vi "Sweep Control.vi"(0 "Scan control":T6=[{"Priority"=enum."Priority 1", "Scan name"=enum."OFF"}, {"Priority"=enum."Priority 0", "Scan name"=enum."Field"}, {"Priority"=enum."Priority 3", "Scan name"=enum."OFF"}, {"Priority"=enum."Priority 2", "Scan name"=enum."OFF"}], 1 "Scan parameters":T4=[{"DAQ Channel"=0, "Label"="\nappliedDC=", "Start"=-0.00372, "End"=0.00428, "Step"=5e-05, "B sweep rate"=0.0}, {"DAQ Channel"=3, "Label"="\nappliedField=", "Start"=0.3, "End"=0.0, "Step"=0.02, "B sweep rate"=0.05}, {"DAQ Channel"=3, "Label"="\nappliedVbg=", "Start"=-1.55, "End"=3.0, "Step"=0.015, "B sweep rate"=2.0}, {"DAQ Channel"=3, "Label"="\nappliedField=", "Start"=0.0, "End"=10000.0, "Step"=5000.0, "B sweep rate"=0.0}] {"B sweep rate" format="%.2f"; "Step" format="%#_6p"; "End" format="%#_6p"; "Start" format="%#_6p"}, 3 "Comments":string="B sweep from 0.3T to 0T, 0.02T step\nDC sweep from -4mV to 4mV, 5uV step\nVbg = -5V\nVsg=40mV\nT<60mK\n\nI+/-: rightwire 1/2 200uV + DC sweep, f=9\nI2-: grounded on 4\nBase f=3\nV+/-: 5/7\nV2+/-: 4/28\nVsg: 6", 4 "Experiment folder name":string="21-SmallBsweep-DCsweep-rightdrive12-leftgrounded") -> ()   [LabVIEW 2016]
uses:
  Typedefs/ScanControl.ctl
  Typedefs/Cluster - ScanControl.ctl
  Typedefs/Enum - Priority.ctl
  Typedefs/Enum - Action.ctl
  Typedefs/ScanParamters.ctl
  Typedefs/Cluster - ScanParamters.ctl
  Typedefs/PostAction.ctl
  Typedefs/Enum - PostAction.ctl
  <userlib>/_OpenG.lib/array/array.llb/Empty 1D Array (Variant)__ogtk.vi
panel:
  in  "Channels: AO":T1={"AO amp (V)"=[0.0002, 0.0, 0.0, 0.0, 0.0, 0.0, 0.0, 0.0], "AO DC (V)"=[-0.004, 0.0, 0.04, 0.0, 0.0, 0.0, 0.0, 0.0], "AO f (Hz)"=[9.0, 3.0, 3.0, 3.0, 3.0, 3.0, 3.0, 3.0], "AO phi (deg)"=[0.0, 0.0, 0.0, 0.0, 0.0, 0.0, 0.0, 0.0], "function"=[enum."Sine Wave", enum."Sine Wave", enum."Sine Wave", enum."Sine Wave", enum."Sine Wave", enum."Sine Wave", enum."Sine Wave", enum."Sine Wave"]} {"AO DC (V)" format="%#_6p"; "AO amp (V)" format="%#_6p"}
  in  "Experiment":enum16{"IV", "lockin_time", "Lockin_Vsg"}(ring)=enum."Lockin_Vsg"
  in  "Post action (indexing priority)":T2=[enum."Do Nothing", enum."Wait", enum."Do Nothing", enum."Do Nothing"]
  in  "Number of IV curves":i32=1
  # "Instructions: \n1, you can put multiple scan names in one priority.\n2 OFF has to put in last priority"
  # "if you use the lockin\nprogram remember to\nset BG/SG parameters in\n'lockin_Vsg_multichannel.vi'"
  # "0"
  # "1"
  # "2"
  # "3"
  # "4"
  # "5"
  # "6"
  # "7"
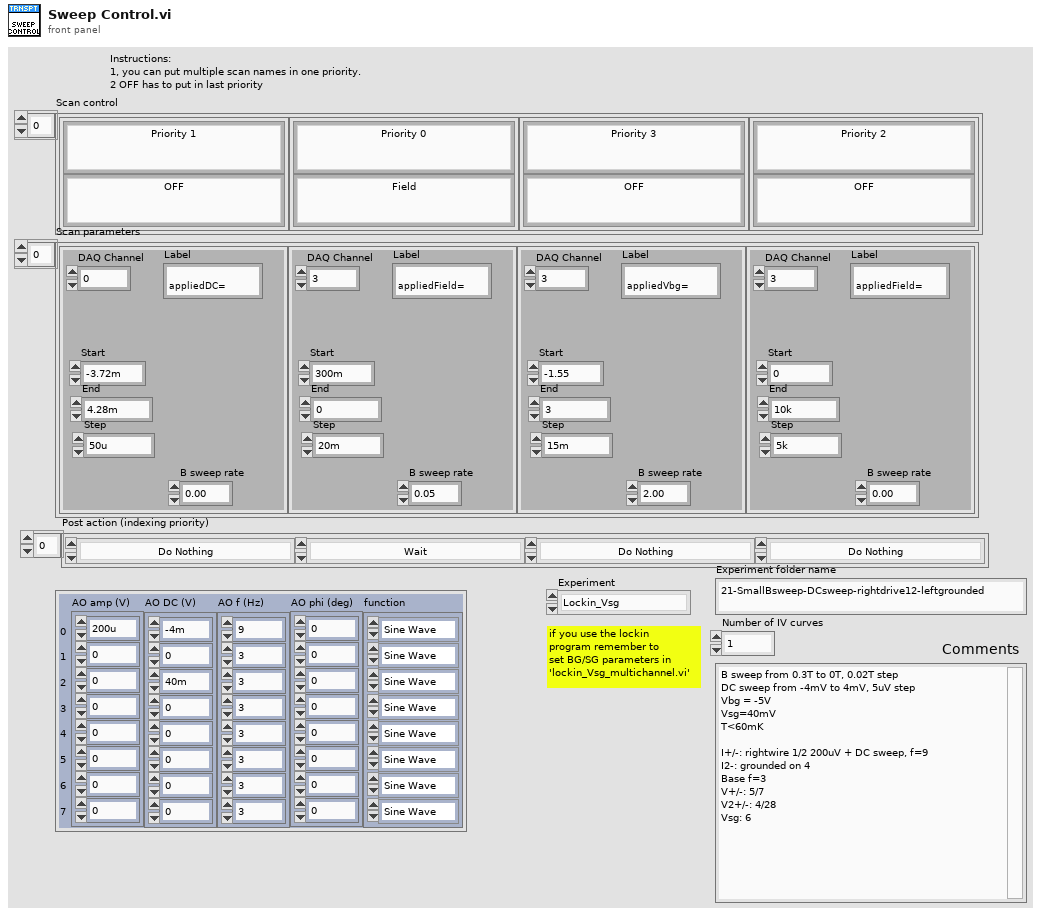
[diagram p1: front panel]
types:
  T1 = cluster{"AO amp (V)":dbl[], "AO DC (V)":dbl[], "AO f (Hz)":dbl[], "AO phi (deg)":dbl[], "function":enum16{"Sine Wave", "Triangle Wave", "Square Wave", "Sawtooth Wave"}[]}
  T2 = typedef "PostAction.ctl" = T3[]
  T3 = typedef "Enum - PostAction.ctl" = enum16{"Clear DAQ Tasks", "Check Temperature", "Wait", "Do Nothing"}
  T4 = typedef "ScanParamters.ctl" = T5[]
  T5 = typedef "Cluster - ScanParamters.ctl" = cluster{"DAQ Channel":i32, "Label":string, "Start":dbl, "End":dbl, "Step":dbl, "B sweep rate":dbl}
  T6 = typedef "ScanControl.ctl" = T7[]
  T7 = typedef "Cluster - ScanControl.ctl" = cluster{"Priority":T8, "Scan name":T9}
  T8 = typedef "Enum - Priority.ctl" = enum16{"Priority 0", "Priority 1", "Priority 2", "Priority 3", "Priority 4", "Priority 5"}
  T9 = typedef "Enum - Action.ctl" = enum16{"OFF", "Vsg1", "Vsg2", "Vsgw", "Vbg", "Vamp", "Field", "Temp", "MW_freq", "MW_amplitude"}
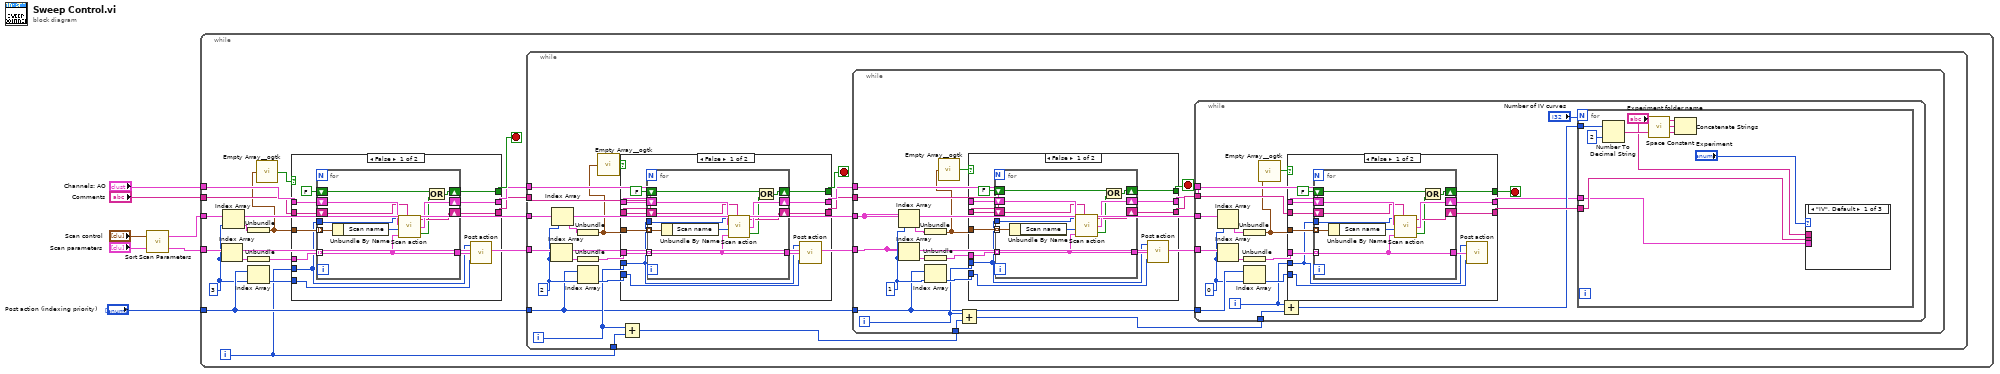
[diagram p0: block diagram]
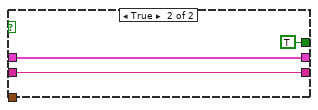
[diagram p2: hidden frame]
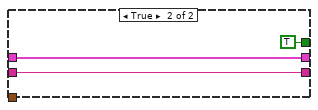
[diagram p3: hidden frame]
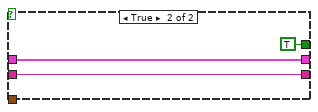
[diagram p4: hidden frame]
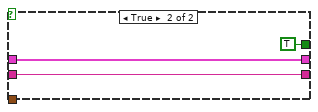
[diagram p5: hidden frame]
diagram:
  n1 = call "Sort Scan Parameters.vi"("Scan parameters"="Scan parameters", "Scan control"="Scan control") -> ("Sorted scan parameters"=w3:cluster{T4}[], "Sorted scan control"=w4:cluster{T6}[])
  n2 = while {
    tunnel: "Comments" -> [w14]
    tunnel: "Channels: AO" -> [w15]
    tunnel: w3 -> [w21]
    tunnel: w4 -> [w20]
    tunnel: "Post action (indexing priority)" -> [w16]
    i -> [w10]
    stop <- w18 stop-if-true
    w11 = 3
    n3 = Index Array(array=w21, index=w11) -> (element=w22:cluster{T4})
    n4 = Index Array(array=w20, index=w11) -> (element=w19:cluster{T6})
    n5 = Unbundle(w19) -> (w8:T6)
    n6 = Unbundle(w22) -> (w23:T4)
    n7 = Index Array(array=w16, index=w11) -> (element=w17:T3)
    n8 = call-poly <userlib>:"Empty Array__ogtk.vi"("Array"=w8) -> ("Empty Array?"=w9:bool)  [unwired: 8 in]
    n9 = case shown="False" w9 {
      tunnel: w23 -> [w34 _]
      tunnel: [w33 w47] -> w13
      tunnel: [w32 w46] -> w12
      tunnel: [w27 TRUE ("Stop?")] -> w18
      tunnel: w8 -> [w31 _]
      tunnel: w10 -> [w29 _]
      tunnel: w17 -> [w24 _]
      tunnel: w15 -> [w26 w47]
      tunnel: w14 -> [w25 w46]
      frame False {
        n10 = for {
          tunnel: w31 -> [w45] mode=indexing
          tunnel: w34 -> [w38] mode=indexing
          tunnel: w29 -> [w39]
          shift-right: [w43] -> w33
          shift-left: w26 -> [w42]
          shift-right: [w41] -> w32
          shift-left: w25 -> [w40]
          tunnel: [w38] -> w30
          shift-right: [w35] -> w27
          shift-left: FALSE -> [w37]
          n11 = Unbundle By Name(w45) -> ("Scan name"=w44:T9)
          n12 = call "Scan action.vi"("Index"=w39, "Channels: AO"=w42, "Scan control"=w44, "Scan Parameters"=w38, "Comments"=w40) -> ("Comments out"=w41:string, "Channels: AO"=w43:T1, "Stop?"=w36:bool)
          n13 = Or(x=w37, y=w36) -> (x .or. y?=w35:bool)
        }
        n14 = call "Post action.vi"("PostAction"=w24, "Scan Parameters"=w30, "Index"=w29) -> ()  [unwired: 1 in]
      }
      frame True {
      }
    }
    n15 = while {
      tunnel: w21 -> [w62]
      tunnel: w20 -> [w61]
      tunnel: w16 -> [w49]
      tunnel: w12 -> [w60]
      tunnel: w13 -> [w59]
      tunnel: w10 -> [w53]
      i -> [w54]
      stop <- w58 stop-if-true
      w55 = 2
      n16 = Index Array(array=w62, index=w55) -> (element=w65:cluster{T4})
      n17 = Index Array(array=w61, index=w55) -> (element=w66:cluster{T6})
      n18 = Unbundle(w66) -> (w50:T6)
      n19 = Unbundle(w65) -> (w64:T4)
      n20 = Index Array(array=w49, index=w55) -> (element=w63:T3)
      n21 = call-poly <userlib>:"Empty Array__ogtk.vi"("Array"=w50) -> ("Empty Array?"=w51:bool)  [unwired: 8 in]
      n22 = case shown="False" w51 {
        tunnel: w64 -> [w77 _]
        tunnel: w59 -> [w76 w91]
        tunnel: w60 -> [w75 w90]
        tunnel: [w74 w91] -> w57
        tunnel: [w73 w90] -> w56
        tunnel: [w67 TRUE ("Stop?")] -> w58
        tunnel: w50 -> [w72 _]
        tunnel: w54 -> [w69 _]
        tunnel: w63 -> [w70 _]
        frame False {
          n23 = for {
            tunnel: w72 -> [w88] mode=indexing
            tunnel: w77 -> [w81] mode=indexing
            tunnel: w69 -> [w82]
            shift-right: [w86] -> w74
            shift-left: w76 -> [w85]
            shift-right: [w84] -> w73
            shift-left: w75 -> [w83]
            tunnel: [w81] -> w71
            shift-right: [w78] -> w67
            shift-left: FALSE -> [w80]
            n24 = Unbundle By Name(w88) -> ("Scan name"=w87:T9)
            n25 = call "Scan action.vi"("Index"=w82, "Channels: AO"=w85, "Scan control"=w87, "Scan Parameters"=w81, "Comments"=w83) -> ("Comments out"=w84:string, "Channels: AO"=w86:T1, "Stop?"=w79:bool)
            n26 = Or(x=w80, y=w79) -> (x .or. y?=w78:bool)
          }
          n27 = call "Post action.vi"("PostAction"=w70, "Scan Parameters"=w71, "Index"=w69) -> ()  [unwired: 1 in]
        }
        frame True {
        }
      }
      n28 = Add(x=w54, y=w53) -> (x+y=w52:i32)
      n29 = while {
        tunnel: w57 -> [w96]
        tunnel: w56 -> [w105]
        tunnel: w61 -> [w104]
        tunnel: w62 -> [w95]
        tunnel: w49 -> [w92]
        tunnel: w52 -> [w98]
        i -> [w99]
        stop <- w101 stop-if-true
        w100 = 1
        n30 = Index Array(array=w104, index=w100) -> (element=w106:cluster{T6})
        n31 = Index Array(array=w95, index=w100) -> (element=w107:cluster{T4})
        n32 = Unbundle(w106) -> (w93:T6)
        n33 = Unbundle(w107) -> (w108:T4)
        n34 = Index Array(array=w92, index=w100) -> (element=w109:T3)
        n35 = call-poly <userlib>:"Empty Array__ogtk.vi"("Array"=w93) -> ("Empty Array?"=w94:bool)  [unwired: 8 in]
        n36 = Add(x=w99, y=w98) -> (x+y=w97:i32)
        n37 = case shown="False" w94 {
          tunnel: w108 -> [w120 _]
          tunnel: w96 -> [w119 w134]
          tunnel: w105 -> [w118 w133]
          tunnel: [w117 w134] -> w102
          tunnel: [w116 w133] -> w103
          tunnel: [w110 TRUE ("Stop?")] -> w101
          tunnel: w93 -> [w115 _]
          tunnel: w99 -> [w112 _]
          tunnel: w109 -> [w113 _]
          frame False {
            n38 = for {
              tunnel: w115 -> [w131] mode=indexing
              tunnel: w120 -> [w124] mode=indexing
              tunnel: w112 -> [w125]
              shift-right: [w129] -> w117
              shift-left: w119 -> [w128]
              shift-right: [w127] -> w116
              shift-left: w118 -> [w126]
              tunnel: [w124] -> w114
              shift-right: [w121] -> w110
              shift-left: FALSE -> [w123]
              n39 = Unbundle By Name(w131) -> ("Scan name"=w130:T9)
              n40 = call "Scan action.vi"("Index"=w125, "Channels: AO"=w128, "Scan control"=w130, "Scan Parameters"=w124, "Comments"=w126) -> ("Comments out"=w127:string, "Channels: AO"=w129:T1, "Stop?"=w122:bool)
              n41 = Or(x=w123, y=w122) -> (x .or. y?=w121:bool)
            }
            n42 = call "Post action.vi"("PostAction"=w113, "Scan Parameters"=w114, "Index"=w112) -> ()  [unwired: 1 in]
          }
          frame True {
          }
        }
        n43 = while {
          tunnel: w104 -> [w152]
          tunnel: w95 -> [w151]
          tunnel: w102 -> [w147]
          tunnel: w103 -> [w146]
          tunnel: w92 -> [w143]
          tunnel: w97 -> [w139]
          i -> [w140]
          stop <- w144 stop-if-true
          w142 = 0
          n44 = Index Array(array=w152, index=w142) -> (element=w150:cluster{T6})
          n45 = Index Array(array=w151, index=w142) -> (element=w149:cluster{T4})
          n46 = Unbundle(w150) -> (w135:T6)
          n47 = Unbundle(w149) -> (w148:T4)
          n48 = Index Array(array=w143, index=w142) -> (element=w141:T3)
          n49 = call-poly <userlib>:"Empty Array__ogtk.vi"("Array"=w135) -> ("Empty Array?"=w136:bool)  [unwired: 8 in]
          n50 = Add(x=w140, y=w139) -> (x+y=w138:i32)
          n51 = case shown="False" w136 {
            tunnel: w148 -> [w164 _]
            tunnel: w147 -> [w163 w178]
            tunnel: w146 -> [w162 w177]
            tunnel: [w161 w178] -> w137
            tunnel: [w160 w177] -> w145
            tunnel: [w155 TRUE ("Stop?")] -> w144
            tunnel: w135 -> [w159 _]
            tunnel: w140 -> [w154 _]
            tunnel: w141 -> [w157 _]
            frame False {
              n52 = for {
                tunnel: w159 -> [w175] mode=indexing
                tunnel: w164 -> [w168] mode=indexing
                tunnel: w154 -> [w169]
                shift-right: [w173] -> w161
                shift-left: w163 -> [w172]
                shift-right: [w171] -> w160
                shift-left: w162 -> [w170]
                tunnel: [w168] -> w158
                shift-right: [w165] -> w155
                shift-left: FALSE -> [w167]
                n53 = Unbundle By Name(w175) -> ("Scan name"=w174:T9)
                n54 = call "Scan action.vi"("Index"=w169, "Channels: AO"=w172, "Scan control"=w174, "Scan Parameters"=w168, "Comments"=w170) -> ("Comments out"=w171:string, "Channels: AO"=w173:T1, "Stop?"=w166:bool)
                n55 = Or(x=w167, y=w166) -> (x .or. y?=w165:bool)
              }
              n56 = call "Post action.vi"("PostAction"=w157, "Scan Parameters"=w158, "Index"=w154) -> ()  [unwired: 1 in]
            }
            frame True {
            }
          }
          n57 = for {
            N: "Number of IV curves" -> [_]
            tunnel: w137 -> [w179]
            tunnel: w145 -> [w181]
            tunnel: w138 -> [w185]
            n58 = Number To Decimal String(number=w185, width (-)=i16 2) -> (decimal integer string=w184:string)
            n59 = call <vilib>:"Space Constant.vi"() -> ("String"=w183:string)
            n60 = Concatenate Strings("Experiment folder name", w183, w184) -> ()  [unwired: 1 out]
            n61 = case shown="\"IV\", Default" "Experiment" {
              tunnel: w181 -> [_ _ _]
              tunnel: "Experiment folder name" -> [_ _ _]
              tunnel: w179 -> [_ _ _]
              frame "IV", Default {
              }
              frame "lockin_time" {
              }
              frame "Lockin_Vsg" {
              }
            }
          }
        }
      }
    }
  }
